vi "Periodic Tasks.vi"(8 "error in":errorcluster) -> ()   [LabVIEW 2017]
doc: "This VI runs in parallel to other robot code. It can contain as many user-defined periodic loops as you need. These can carry out PID or other sorts of timed response."
uses:
  VIs/CtrlRefs/DioDisplayALB.ctl
  VIs/CtrlRefs/SettingsALB.ctl
  <vilib>/Rock Robotics/WPI/Utilities/WPI_GetSetVariantRefNum.vi
  Robot Global Data.vi
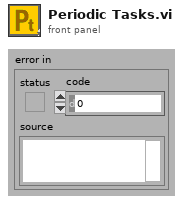
[diagram p1: front panel]
types:
  T1 = typedef "WPI_JoystickDevRef.ctl" = cluster{"Device":T2}
  T2 = typedef "WPI_JoystickDeviceEnum.ctl" = enum16{"USB 0", "USB 1", "USB 2", "USB 3", "USB 4", "USB 5"}
  T3 = typedef "SettingsALB.ctl" = cluster{"Unused 1":dbl, "Unused 2":dbl, "Unused 3":dbl, "Unused 4":dbl, "Unused 5":dbl, "Unused 6":dbl, "Unused 7":dbl, "Unused 8":dbl, "Unused 9":dbl, "Unused 10":dbl, "Unused 11":dbl, "Unused 12":dbl}
  T4 = typedef "WPI_SwitchDevRef.ctl" = cluster{"DevStatus":errorcluster, "DIO Channel":T5, "CntIndex":T6, "Normally Closed":bool}
  T5 = typedef "FPGA_DIOChannel.ctl" = enum8{"DIO 0", "DIO 1", "DIO 2", "DIO 3", "DIO 4", "DIO 5", "DIO 6", "DIO 7", "DIO 8", "DIO 9", "DIO MXP 0", "DIO MXP 1", "DIO MXP 2", "DIO MXP 3", "DIO MXP 4", "DIO MXP 5", "DIO MXP 6", "DIO MXP 7", "DIO MXP 8", "DIO MXP 9", "DIO MXP 10", "DIO MXP 11", "DIO MXP 12", "DIO MXP 13", "DIO MXP 14", "DIO MXP 15", "SPI Port CS1", "SPI Port CS2", "SPI Port CS3", "SPI Port MISO", "SPI Port MOSI", "Invalid"}
  T6 = typedef "FPGA_CounterCtrSystemIndex.ctl" = enum8{"Ctr 0", "Ctr 1", "Ctr 2", "Ctr 3", "Ctr 4", "Ctr 5", "Ctr 6", "Ctr 7", "Invalid"}
  T7 = enum16{"initialize", "read", "write", "write all"}
  T8 = typedef "DioDisplayALB.ctl" = cluster{"DIO 0-LiftMinLimitSwitch":bool, "DIO 1-LiftMaxLimitSwitch":bool, "DIO 2-LiftArmMinLimitSwitch":bool, "DIO 3-LiftArmMaxLimitSwitch":bool, "DIO 4-RightArmMaxLimitSwitch":bool, "DIO 5-RightArmMinLimitSwitch":bool, "DIO 6-LeftArmMaxLimitSwitch":bool, "DIO 7-LeftArmMinLimitSwitch":bool, "DIO 8":bool, "DIO 9":bool}
  T9 = cluster{"LX_Axis":dbl, "LY_Axis":dbl, "LTrigger_Axis":dbl, "RTrigger_Axis":dbl, "RX_Axis":dbl, "RY_Axis":dbl, "Button_0":bool, "Button_1":bool, "Button_2":bool, "Button_3":bool, "Button_4":bool, "Button_5":bool, "Button_6":bool, "Button_7":bool, "Button_8":bool, "Button_9":bool, "POV_0":i16, "POV_1":i16}
  T10 = cluster{"upper limit":dbl, "upper limit":dbl, "upper limit":dbl, "upper limit":dbl, "upper limit":dbl, "upper limit":dbl, bool, bool, bool, bool, bool, bool, bool, bool, bool, bool}
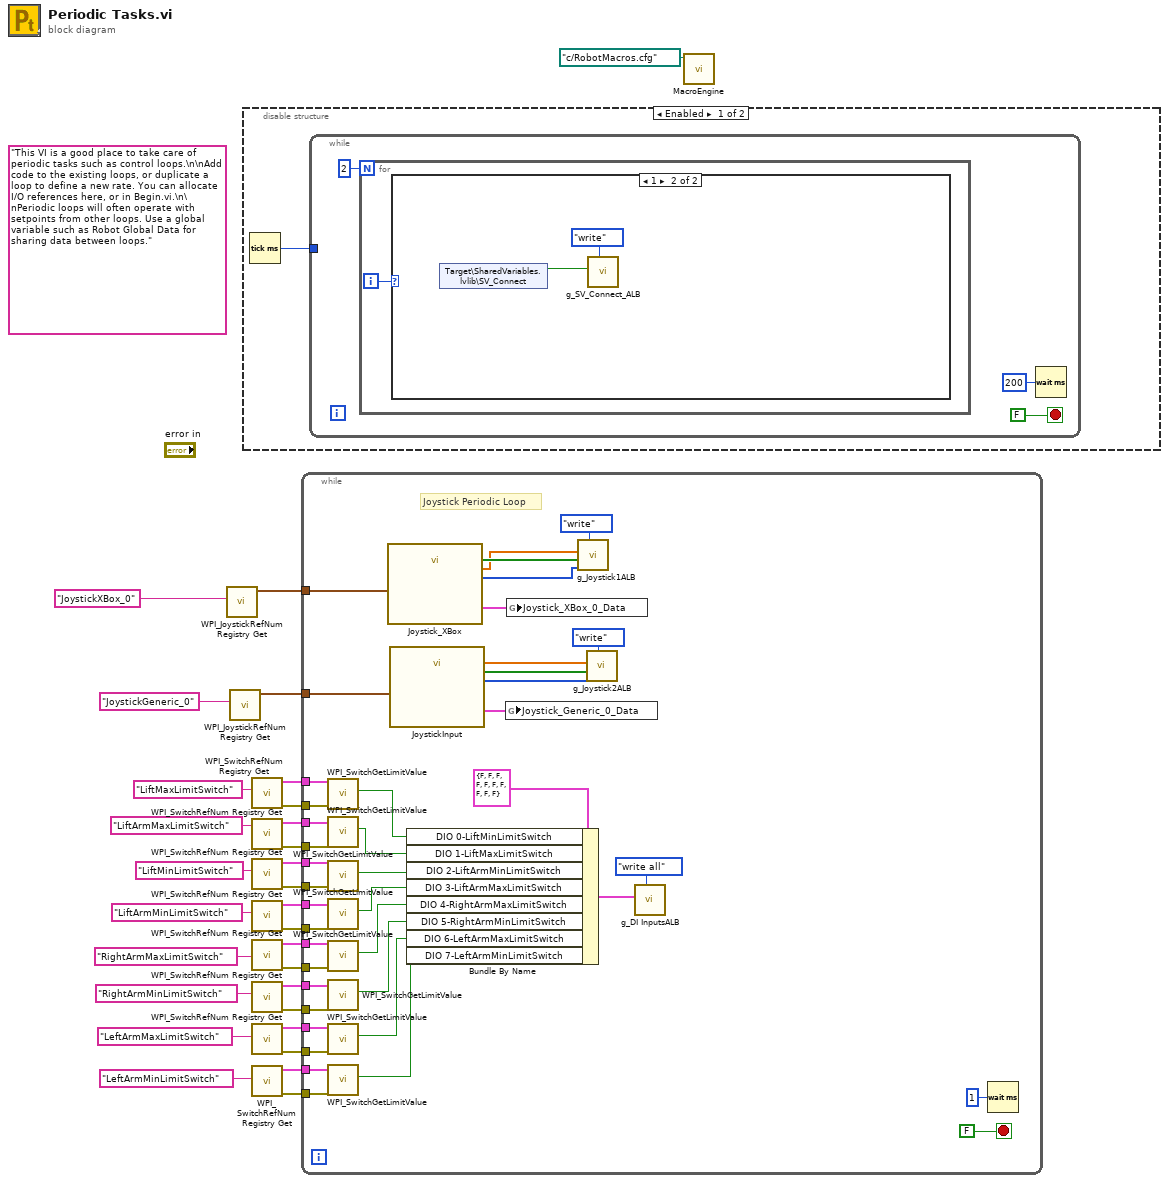
[diagram p0: block diagram]
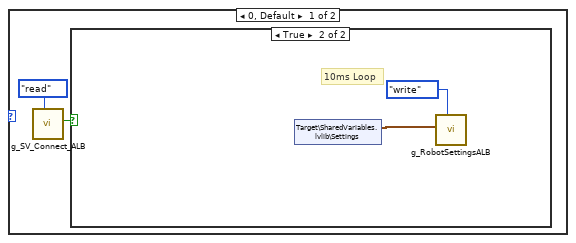
[diagram p2: hidden frame]
diagram:
  (unwired) "This VI is a good place to take care of periodic tasks such as control loops.\n\nAdd code to the existing loops, or duplicate a loop to define a new rate. You can allocate I/O references here, or in Begin.vi.\n\nPeriodic loops will often operate with setpoints from other loops. Use a global variable such as Robot Global Data for sharing data between loops."
  n1 = call <vilib>:"WPI_JoystickRefNum Registry Get.vi"("refnum name"="JoystickXBox_0") -> ("JoystickDevRef"=w3:T1)  [unwired: 9 in, 1 out]
  n2 = call <vilib>:"WPI_JoystickRefNum Registry Get.vi"("refnum name"="JoystickGeneric_0") -> ("JoystickDevRef"=w1:T1)  [unwired: 9 in, 1 out]
  n3 = disable-structure shown="Enabled" {
    frame Enabled {
      n4 = Tick Count (ms)() -> (millisecond timer value=w30:u32)
      n5 = while {
        tunnel: w30 -> [_]
        stop <- FALSE stop-if-true
        n6 = for {
          N: 2 -> [_]
          i -> [w34]
          n7 = case shown="1" w34 {
            frame 0, Default {
              n8 = call "g_SV_Connect_ALB.vi"("Action"=enum16{"read", "write"}."read") -> ("Connected"=w35:bool)  [unwired: 10 in]
              n9 = case shown="True" w35 {
                frame False {
                }
                frame True {
                  # "10ms Loop"
                  n10 = shared-variable "Target\\SharedVariables.lvlib\\Settings"() -> (w37:T3)  [unwired: 1 in, 1 out]
                  n11 = call "g_RobotSettingsALB.vi"("Action"=enum16{"read", "write"}."write", "Settings"=w37) -> ()  [unwired: 9 in, 1 out]
                }
              }
            }
            frame 1 {
              n12 = shared-variable "Target\\SharedVariables.lvlib\\SV_Connect"() -> (w39:bool)  [unwired: 1 in, 1 out]
              n13 = call "g_SV_Connect_ALB.vi"("Action"=enum16{"read", "write"}."write", "Connect in"=w39) -> ()  [unwired: 9 in, 1 out]
            }
          }
        }
        n14 = Wait (ms)(milliseconds to wait=u32 200) -> ()  [unwired: 1 out]
      }
    }
    frame Disabled {
    }
  }
  n15 = call <vilib>:"WPI_SwitchRefNum Registry Get.vi"("refnum name"="LiftMaxLimitSwitch") -> ("error out"=w17:errorcluster, "SwitchDevRef"=w21:T4)  [unwired: 9 in]
  n16 = call <vilib>:"WPI_SwitchRefNum Registry Get.vi"("refnum name"="LiftArmMaxLimitSwitch") -> ("error out"=w16:errorcluster, "SwitchDevRef"=w20:T4)  [unwired: 9 in]
  n17 = call <vilib>:"WPI_SwitchRefNum Registry Get.vi"("refnum name"="LiftMinLimitSwitch") -> ("error out"=w6:errorcluster, "SwitchDevRef"=w19:T4)  [unwired: 9 in]
  n18 = call <vilib>:"WPI_SwitchRefNum Registry Get.vi"("refnum name"="LiftArmMinLimitSwitch") -> ("error out"=w15:errorcluster, "SwitchDevRef"=w18:T4)  [unwired: 9 in]
  n19 = call <vilib>:"WPI_SwitchRefNum Registry Get.vi"("refnum name"="RightArmMaxLimitSwitch") -> ("error out"=w14:errorcluster, "SwitchDevRef"=w13:T4)  [unwired: 9 in]
  n20 = call <vilib>:"WPI_SwitchRefNum Registry Get.vi"("refnum name"="RightArmMinLimitSwitch") -> ("error out"=w11:errorcluster, "SwitchDevRef"=w12:T4)  [unwired: 9 in]
  n21 = call <vilib>:"WPI_SwitchRefNum Registry Get.vi"("refnum name"="LeftArmMaxLimitSwitch") -> ("error out"=w9:errorcluster, "SwitchDevRef"=w10:T4)  [unwired: 9 in]
  n22 = call <vilib>:"WPI_SwitchRefNum Registry Get.vi"("refnum name"="LeftArmMinLimitSwitch") -> ("error out"=w7:errorcluster, "SwitchDevRef"=w8:T4)  [unwired: 9 in]
  n23 = while {
    tunnel: w3 -> [w77]
    tunnel: w1 -> [w79]
    tunnel: w21 -> [w62]
    tunnel: w20 -> [w60]
    tunnel: w19 -> [w68]
    tunnel: w18 -> [w58]
    tunnel: w17 -> [w61]
    tunnel: w16 -> [w69]
    tunnel: w15 -> [w67]
    tunnel: w14 -> [w66]
    tunnel: w13 -> [w57]
    tunnel: w12 -> [w56]
    tunnel: w11 -> [w65]
    tunnel: w10 -> [w55]
    tunnel: w9 -> [w64]
    tunnel: w8 -> [w54]
    tunnel: w7 -> [w63]
    tunnel: w6 -> [w59]
    stop <- FALSE stop-if-true
    # "Joystick Periodic Loop"
    n24 = call <vilib>:"WPI_SwitchGetLimitValue.vi"("error in (no error)"=w61, "SwitchDevRef"=w62) -> ("Switch Pressed"=w53:bool)  [unwired: 7 in, 2 out]
    n25 = call <vilib>:"WPI_SwitchGetLimitValue.vi"("error in (no error)"=w69, "SwitchDevRef"=w60) -> ("Switch Pressed"=w49:bool)  [unwired: 7 in, 2 out]
    n26 = call <vilib>:"WPI_SwitchGetLimitValue.vi"("error in (no error)"=w59, "SwitchDevRef"=w68) -> ("Switch Pressed"=w48:bool)  [unwired: 7 in, 2 out]
    n27 = call <vilib>:"WPI_SwitchGetLimitValue.vi"("error in (no error)"=w67, "SwitchDevRef"=w58) -> ("Switch Pressed"=w47:bool)  [unwired: 7 in, 2 out]
    n28 = call <vilib>:"WPI_SwitchGetLimitValue.vi"("error in (no error)"=w66, "SwitchDevRef"=w57) -> ("Switch Pressed"=w46:bool)  [unwired: 7 in, 2 out]
    n29 = call <vilib>:"WPI_SwitchGetLimitValue.vi"("error in (no error)"=w65, "SwitchDevRef"=w56) -> ("Switch Pressed"=w45:bool)  [unwired: 7 in, 2 out]
    n30 = call <vilib>:"WPI_SwitchGetLimitValue.vi"("error in (no error)"=w64, "SwitchDevRef"=w55) -> ("Switch Pressed"=w44:bool)  [unwired: 7 in, 2 out]
    n31 = call <vilib>:"WPI_SwitchGetLimitValue.vi"("error in (no error)"=w63, "SwitchDevRef"=w54) -> ("Switch Pressed"=w43:bool)  [unwired: 7 in, 2 out]
    n32 = call "Joystick_XBox.vi"("JoystickDevRef"=w77) -> ("Generic_Axes"=w73:dbl[], "Generic_Buttons"=w74:bool[], "Joystick_XBox"=w76:T9, "POVs"=w41:i16[])  [unwired: 7 in]
    n33 = call "JoystickInput.vi"("JoystickDevRef"=w79) -> ("Buttons"=w70:bool[], "Axes"=w72:dbl[], "output cluster"=w78:T10, "POVs"=w42:i16[])  [unwired: 7 in]
    n34 = Bundle By Name(cluster=T8 {"DIO 0-LiftMinLimitSwitch"=FALSE, "DIO 1-LiftMaxLimitSwitch"=FALSE, "DIO 2-LiftArmMinLimitSwitch"=FALSE, "DIO 3-LiftArmMaxLimitSwitch"=FALSE, "DIO 4-RightArmMaxLimitSwitch"=FALSE, "DIO 5-RightArmMinLimitSwitch"=FALSE, "DIO 6-LeftArmMaxLimitSwitch"=FALSE, "DIO 7-LeftArmMinLimitSwitch"=FALSE, "DIO 8"=FALSE, "DIO 9"=FALSE} ("DI All in"), "DIO 0-LiftMinLimitSwitch"=w53, "DIO 1-LiftMaxLimitSwitch"=w49, "DIO 2-LiftArmMinLimitSwitch"=w48, "DIO 3-LiftArmMaxLimitSwitch"=w47, "DIO 4-RightArmMaxLimitSwitch"=w46, "DIO 5-RightArmMinLimitSwitch"=w45, "DIO 6-LeftArmMaxLimitSwitch"=w44, "DIO 7-LeftArmMinLimitSwitch"=w43) -> (w50:T8)
    n35 = global write "Robot Global Data.vi" "Joystick_Generic_0_Data"(w78) -> ()
    n36 = global write "Robot Global Data.vi" "Joystick_XBox_0_Data"(w76) -> ()
    n37 = call "g_Joystick1ALB.vi"("Action"=enum16{"initialize", "read", "write"}."write", "POVs"=w41, "Buttons"=w74, "Axes"=w73) -> ()  [unwired: 4 in, 4 out]
    n38 = call "g_Joystick2ALB.vi"("Action"=enum16{"initialize", "read", "write"}."write", "POVs"=w42, "Buttons"=w70, "Axes"=w72) -> ()  [unwired: 4 in, 4 out]
    n39 = call "g_DI InputsALB.vi"("Action"=T7."write all", "DI All in"=w50) -> ()  [unwired: 9 in, 1 out]
    n40 = Wait (ms)(milliseconds to wait=u32 1) -> ()  [unwired: 1 out]
  }
  n41 = call "MacroEngine.vi"("File Path"=path "c:/RobotMacros.cfg") -> ()  [unwired: 11 in]
